vi "OCR_Build Bit Line Array.vi"(8 "Error":errorcluster, 11 "2D Image":T7=[[255, 255, 255, 255, 255, 255, 255, 255, 255, 255, 255, 255, 255, 255, 255, 255, 255, 255, 255, 255, 255, 255, 255, 255, 255, 255, 255, 255, 255, 255, 255, 255], [255, 255, 255, 255, 255, 255, 16776960, 16776960, 16776960, 255, 255, 16776960, 16776960, 255, 255, 255, 16776960, 16776960, 16776960, 255, 255, 16776960, 255, 255, 255, 16776960, 255, 255, 255, 255, 255, 255], [255, 255, 255, 255, 255, 255, 255, 16776960, 255, 255, 16776960, 255, 255, 16776960, 255, 16776960, 255, 255, 255, 16776960, 255, 16776960, 16776960, 255, 255, 16776960, 255, 255, 255, 255, 255, 255], [255, 255, 255, 255, 255, 255, 255, 16776960, 255, 255, 16776960, 255, 255, 255, 255, 16776960, 255, 255, 255, 16776960, 255, 16776960, 255, 16776960, 255, 16776960, 255, 255, 255, 255, 255, 255], [255, 255, 255, 255, 255, 255, 255, 16776960, 255, 255, 16776960, 255, 255, 16776960, 255, 16776960, 255, 255, 255, 16776960, 255, 16776960, 255, 255, 16776960, 16776960, 255, 255, 255, 255, 255, 255], [255, 255, 255, 255, 255, 255, 16776960, 16776960, 16776960, 255, 255, 16776960, 16776960, 255, 255, 255, 16776960, 16776960, 16776960, 255, 255, 16776960, 255, 255, 255, 16776960, 255, 255, 255, 255, 255, 255], [255, 255, 255, 255, 255, 255, 255, 255, 255, 255, 255, 255, 255, 255, 255, 255, 255, 255, 255, 255, 255, 255, 255, 255, 255, 255, 255, 255, 255, 255, 255, 255], [255, 16776960, 16776960, 16776960, 16776960, 16776960, 16776960, 16776960, 16776960, 16776960, 16776960, 16776960, 16776960, 16776960, 16776960, 16776960, 16776960, 16776960, 16776960, 16776960, 16776960, 16776960, 16776960, 16776960, 16776960, 16776960, 16776960, 16776960, 16776960, 16776960, 16776960, 255], [255, 16776960, 16776960, 16776960, 16776960, 16776960, 16776960, 16776960, 16776960, 16776960, 16776960, 16776960, 16776960, 16776960, 16776960, 16776960, 16776960, 16776960, 16776960, 16776960, 16776960, 16776960, 16776960, 16776960, 16776960, 16776960, 16776960, 16776960, 16776960, 16776960, 16776960, 255], [255, 16776960, 16776960, 16776960, 16776960, 16776960, 16776960, 16776960, 16776960, 16776960, 16776960, 16776960, 16776960, 16776960, 16776960, 16776960, 16776960, 16776960, 16776960, 16776960, 16776960, 16776960, 16776960, 16776960, 16776960, 16776960, 16776960, 16776960, 16776960, 16776960, 16776960, 255], [255, 16776960, 16776960, 255, 255, 16776960, 16776960, 255, 255, 255, 16776960, 16776960, 255, 255, 255, 255, 16776960, 16776960, 255, 255, 16776960, 16776960, 255, 255, 255, 16776960, 255, 255, 255, 255, 16776960, 255], [255, 16776960, 255, 16776960, 16776960, 255, 16776960, 255, 16776960, 16776960, 255, 16776960, 255, 16776960, 16776960, 16776960, 16776960, 255, 16776960, 16776960, 255, 16776960, 16776960, 255, 16776960, 16776960, 255, 16776960, 16776960, 16776960, 16776960, 255], [255, 16776960, 255, 16776960, 16776960, 16776960, 16776960, 255, 255, 255, 16776960, 16776960, 255, 255, 255, 16776960, 16776960, 255, 255, 255, 255, 16776960, 16776960, 255, 16776960, 16776960, 255, 255, 255, 16776960, 16776960, 255], [255, 16776960, 255, 16776960, 16776960, 255, 16776960, 255, 16776960, 16776960, 255, 16776960, 255, 16776960, 16776960, 16776960, 16776960, 255, 16776960, 16776960, 255, 16776960, 16776960, 255, 16776960, 16776960, 255, 16776960, 16776960, 16776960, 16776960, 255], [255, 16776960, 16776960, 255, 255, 16776960, 16776960, 255, 16776960, 16776960, 255, 16776960, 255, 255, 255, 255, 16776960, 255, 16776960, 16776960, 255, 16776960, 16776960, 255, 16776960, 16776960, 255, 255, 255, 255, 16776960, 255], [255, 16776960, 16776960, 16776960, 16776960, 16776960, 16776960, 16776960, 16776960, 16776960, 16776960, 16776960, 16776960, 16776960, 16776960, 16776960, 16776960, 16776960, 16776960, 16776960, 16776960, 16776960, 16776960, 16776960, 16776960, 16776960, 16776960, 16776960, 16776960, 16776960, 16776960, 255], [255, 16776960, 16776960, 16776960, 16776960, 16776960, 16776960, 16776960, 16776960, 16776960, 16776960, 16776960, 16776960, 16776960, 16776960, 16776960, 16776960, 16776960, 16776960, 16776960, 16776960, 16776960, 16776960, 16776960, 16776960, 16776960, 16776960, 16776960, 16776960, 16776960, 16776960, 255], [255, 16776960, 16776960, 16776960, 16776960, 16776960, 16776960, 16776960, 16776960, 16776960, 16776960, 16776960, 255, 255, 255, 16776960, 16776960, 255, 255, 255, 16776960, 16776960, 16776960, 16776960, 16776960, 16776960, 16776960, 16776960, 16776960, 16776960, 16776960, 255], [255, 16776960, 16776960, 16776960, 16776960, 16776960, 16776960, 16776960, 16776960, 16776960, 16776960, 16776960, 16776960, 16776960, 16776960, 255, 16776960, 255, 16776960, 16776960, 255, 16776960, 16776960, 16776960, 16776960, 16776960, 16776960, 16776960, 16776960, 16776960, 16776960, 255], [255, 16776960, 16776960, 16776960, 16776960, 16776960, 16776960, 16776960, 16776960, 16776960, 16776960, 16776960, 16776960, 255, 255, 16776960, 16776960, 255, 16776960, 16776960, 255, 16776960, 16776960, 16776960, 16776960, 16776960, 16776960, 16776960, 16776960, 16776960, 16776960, 255], [255, 16776960, 16776960, 16776960, 16776960, 16776960, 16776960, 16776960, 16776960, 16776960, 16776960, 16776960, 255, 16776960, 16776960, 16776960, 16776960, 255, 16776960, 16776960, 255, 16776960, 16776960, 16776960, 16776960, 16776960, 16776960, 16776960, 16776960, 16776960, 16776960, 255], [255, 16776960, 16776960, 16776960, 16776960, 16776960, 16776960, 16776960, 16776960, 16776960, 16776960, 16776960, 255, 255, 255, 255, 16776960, 255, 255, 255, 16776960, 16776960, 16776960, 16776960, 16776960, 16776960, 16776960, 16776960, 16776960, 16776960, 16776960, 255], [255, 16776960, 16776960, 16776960, 16776960, 16776960, 16776960, 16776960, 16776960, 16776960, 16776960, 16776960, 16776960, 16776960, 16776960, 16776960, 16776960, 16776960, 16776960, 16776960, 16776960, 16776960, 16776960, 16776960, 16776960, 16776960, 16776960, 16776960, 16776960, 16776960, 16776960, 255], [255, 16776960, 16776960, 16776960, 16776960, 16776960, 16776960, 16776960, 16776960, 16776960, 16776960, 16776960, 16776960, 16776960, 16776960, 16776960, 16776960, 16776960, 16776960, 16776960, 16776960, 16776960, 16776960, 16776960, 16776960, 16776960, 16776960, 16776960, 16776960, 16776960, 16776960, 255], [255, 16776960, 16776960, 16776960, 16776960, 255, 255, 16776960, 16776960, 255, 255, 255, 16776960, 16776960, 255, 255, 255, 16776960, 16776960, 16776960, 255, 255, 16776960, 16776960, 255, 16776960, 16776960, 16776960, 255, 16776960, 16776960, 255], [255, 16776960, 16776960, 16776960, 255, 16776960, 16776960, 255, 16776960, 255, 16776960, 16776960, 255, 16776960, 255, 16776960, 16776960, 255, 16776960, 255, 16776960, 16776960, 255, 16776960, 16776960, 255, 16776960, 255, 16776960, 16776960, 16776960, 255], [255, 16776960, 16776960, 16776960, 255, 255, 255, 255, 16776960, 255, 255, 255, 16776960, 16776960, 255, 255, 255, 16776960, 16776960, 255, 255, 255, 255, 16776960, 16776960, 16776960, 255, 16776960, 16776960, 16776960, 16776960, 255], [255, 16776960, 16776960, 16776960, 255, 16776960, 16776960, 255, 16776960, 255, 16776960, 16776960, 255, 16776960, 255, 16776960, 16776960, 255, 16776960, 255, 16776960, 16776960, 255, 16776960, 16776960, 16776960, 255, 16776960, 16776960, 16776960, 16776960, 255], [255, 16776960, 16776960, 16776960, 255, 16776960, 16776960, 255, 16776960, 255, 16776960, 16776960, 255, 16776960, 255, 16776960, 16776960, 255, 16776960, 255, 16776960, 16776960, 255, 16776960, 16776960, 16776960, 255, 16776960, 16776960, 16776960, 16776960, 255], [255, 16776960, 16776960, 16776960, 16776960, 16776960, 16776960, 16776960, 16776960, 16776960, 16776960, 16776960, 16776960, 16776960, 16776960, 16776960, 16776960, 16776960, 16776960, 16776960, 16776960, 16776960, 16776960, 16776960, 16776960, 16776960, 16776960, 16776960, 16776960, 16776960, 16776960, 255], [255, 16776960, 16776960, 16776960, 16776960, 16776960, 16776960, 16776960, 16776960, 16776960, 16776960, 16776960, 16776960, 16776960, 16776960, 16776960, 16776960, 16776960, 16776960, 16776960, 16776960, 16776960, 16776960, 16776960, 16776960, 16776960, 16776960, 16776960, 16776960, 16776960, 16776960, 255], [255, 255, 255, 255, 255, 255, 255, 255, 255, 255, 255, 255, 255, 255, 255, 255, 255, 255, 255, 255, 255, 255, 255, 255, 255, 255, 255, 255, 255, 255, 255, 255]]) -> (0 "Error Out":errorcluster, 1 "Text Out":T1[](array[typedef]), 2 "Colors Out":T2, 3 "Format Out":T4={"Rule"=enum."Static", "Header"=TRUE, "Rows"=5, "Width"=32, "Position"=enum."MID-CTR"} {"Rows" min=1 max=5 step=1; "Width" min=7 max=32 step=1}, 4 "Status Of Each Line Out":bool[](array[boolean]))   [LabVIEW 2009]
doc: "Built an array of bit arrays for each line in the 2D Image"
uses:
  Controls/Array/Color Box Array_2D Icon Viewer.ctl
  Controls/Cluster/Cluster_Sizing Data.ctl
  Controls/Enum/ENUM_Icon Sizing.ctl
  Controls/Enum/RBENUM_Icon Position.ctl
  Controls/Cluster/Cluster_Icon Color Set.ctl
  Controls/Enum/ENUM_Frame Template Select.ctl
  Controls/String_Picture/STRING_Line Display.ctl
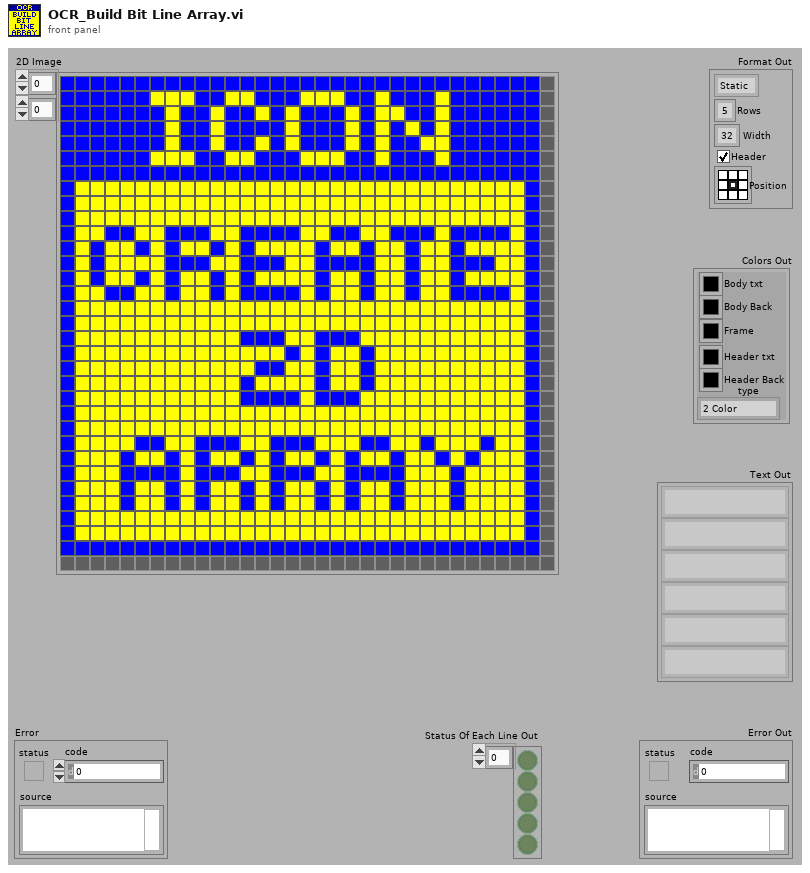
[diagram p1: front panel]
types:
  T1 = typedef "STRING_Line Display.ctl" = string
  T2 = typedef "Cluster_Icon Color Set.ctl" = cluster{"Body txt":u32, "Body Back":u32, "Frame":u32, "Header txt":u32, "Header Back":u32, "type":T3}
  T3 = typedef "ENUM_Frame Template Select.ctl" = enum16{"2 Color", "5 Color"}
  T4 = typedef "Cluster_Sizing Data.ctl" = cluster{"Rule":T5, "Header":bool, "Rows":u32, "Width":u32, "Position":T6}
  T5 = typedef "ENUM_Icon Sizing.ctl" = enum16{"Static", "Auto"}
  T6 = typedef "RBENUM_Icon Position.ctl" = enum32{"LFT-TOP", "MID-TOP", "RGT-TOP", "LFT-CTR", "MID-CTR", "RGT-CTR", "LFT-BOT", "MID-BOT", "RGT-BOT"}
  T7 = typedef "Color Box Array_2D Icon Viewer.ctl" = u32[][]
  T8 = typedef "Cluster_Region info.ctl" = cluster{"Left":i32, "Top":i32, "Right":i32, "Bottom":i32, "Width":u32, "Height":u32, "Start":T9}
  T9 = typedef "Cluster_Top Left position.ctl" = cluster{"Left":i32, "Top":i32}
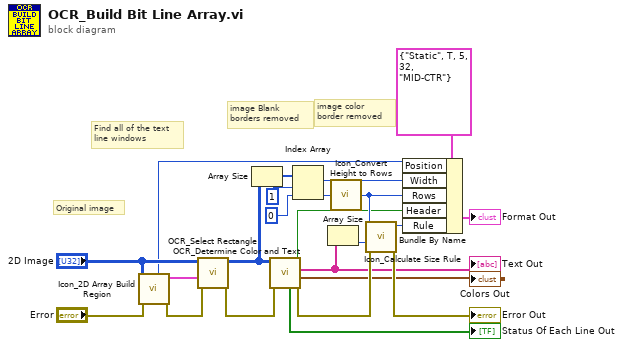
[diagram p0: block diagram]
diagram:
  # "image color\nborder removed"
  # "image Blank\nborders removed"
  # "Original image"
  # "Find all of the text\nline windows"
  n1 = call "Icon_2D Array Build Region.vi"("Error"="Error", "2D Image"="2D Image") -> ("Error Out"=w19:errorcluster, "Region Out"=w18:T8, "Position Out"=w20:T6)  [unwired: 7 in]
  n2 = call "OCR_Select Rectangle.vi"("Error"=w19, "Region"=w18, "2D Image"="2D Image") -> ("Error Out"=w6:errorcluster, "2D Image Out"=w5:T7)  [unwired: 7 in]
  n3 = Array Size(array=w5) -> (size(s)=w14:i32[])
  n4 = call "OCR_Determine Color and Text.vi"("Error"=w6, "Border Removed"=w5) -> ("Error Out"=w7:errorcluster, "Colors Out"=→"Colors Out":T2, "Text Out"=w3:T1[], "Header Out"=w1:bool, "Status Of Each Line Out"=→"Status Of Each Line Out":bool[])  [unwired: 5 in]
  "Text Out" <- w3
  n5 = Index Array(array=w14, index #1=1 ("index"), index #2=0 ("index")) -> (element #1=w11:i32, element #2=w10:i32)
  n6 = Array Size(array=w3) -> (size(s)=w9:i32)
  n7 = call "Icon_Convert Height to Rows.vi"("Height"=w10) -> ("Rows"=w8:u32)  [unwired: 4 in]
  n8 = call "Icon_Calculate Size Rule.vi"("Error"=w7, "Text Size"=w9, "Rows"=w8) -> ("Error Out"=→"Error Out":errorcluster, "Rule Out"=w17:T5)  [unwired: 7 in]
  n9 = Bundle By Name(cluster=T4 {"Rule"=enum."Static", "Header"=TRUE, "Rows"=5, "Width"=32, "Position"=enum."MID-CTR"} ("Format Out"), "Position"=w20, "Width"=w11, "Rows"=w8, "Header"=w1, "Rule"=w17) -> (→"Format Out":T4)
